vi "Find Intersections of Fitted Line with Universal Circle.vi"(8 "Error In":errorcluster, 10 "Complex Coordinates":cluster{"g Array":sgl[], "s Array":sgl[]}, 11 "Phasor Array":T1[](array[typedef]) {"s" format="%#_4g"; "g" format="%#_4g"}) -> (0 "Error Out":errorcluster, 1 "mu-":dbl format="%#_4g", 2 "Intersection 2":cluster{"x":dbl, "y":dbl} {"x" format="%#_4g"; "y" format="%#_4g"}, 3 "Intersection 1":cluster{"x":dbl, "y":dbl} {"x" format="%#_4g"; "y" format="%#_4g"}, 5 "mu+":dbl format="%#_4g")   [LabVIEW 2019]
uses:
  Phasor (g, s).ctl
  <vilib>/Utility/error.llb/DialogType.ctl
  <vilib>/Analysis/6fits.llb/Curve Fitting Criteria.ctl
  <vilib>/Analysis/NI_AALPro.lvlib
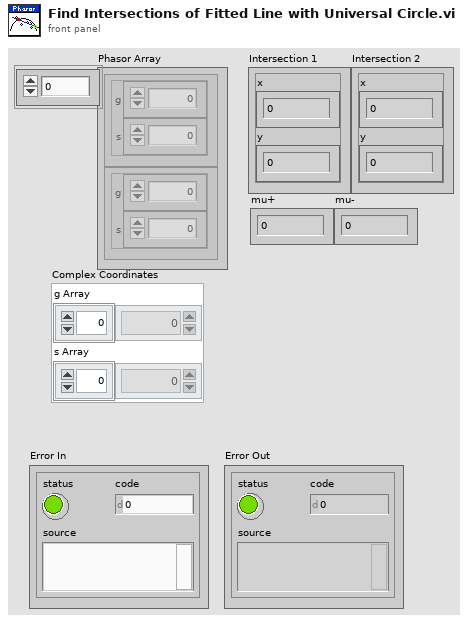
[diagram p1: front panel]
types:
  T1 = typedef "Phasor (g, s).ctl" = cluster{"g":dbl, "s":dbl}
  T2 = typedef "DialogType.ctl" = u16
  T3 = typedef "NI_AALPro.lvlib/Curve Fitting Criteria.ctl" = u16
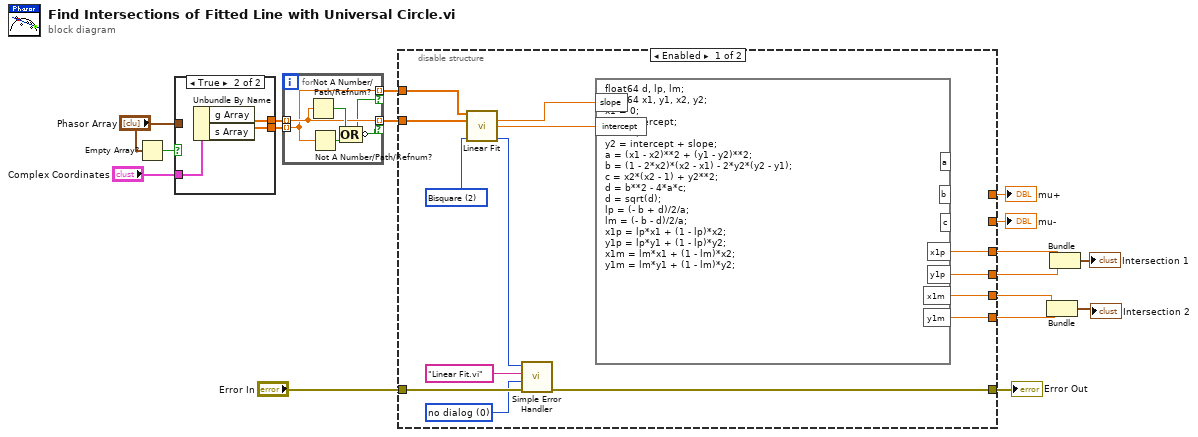
[diagram p0: block diagram]
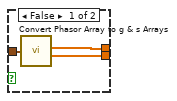
[diagram p2: hidden frame]
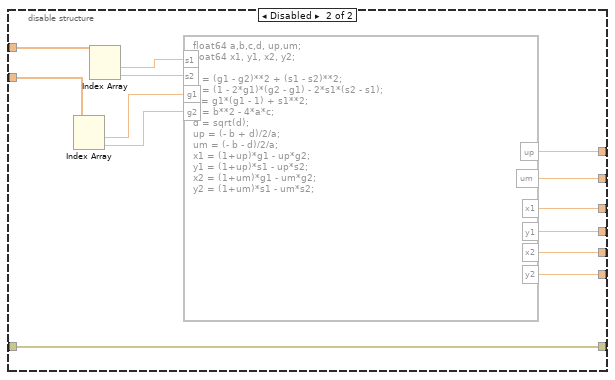
[diagram p3: hidden frame]
diagram:
  n1 = Empty Array?(array="Phasor Array") -> (empty?=w2:bool)
  n2 = case shown="True" w2 {
    tunnel: [w20 w22] -> w9
    tunnel: [w19 w21] -> w8
    tunnel: "Phasor Array" -> [w18 _]
    tunnel: "Complex Coordinates" -> [_ w23]
    frame False {
      n3 = call "Convert Phasor Array to g & s Arrays.vi"("Phasor Array"=w18) -> ("g"=w20:dbl[], "s"=w19:dbl[])  [unwired: 8 in]
    }
    frame True {
      n4 = Unbundle By Name(w23) -> ("g Array"=w22:sgl[], "s Array"=w21:sgl[])
    }
  }
  n5 = for {
    tunnel: w9 -> [w26] mode=indexing
    tunnel: w8 -> [w25] mode=indexing
    tunnel: [w26] -> w7 mode=indexing if=w24
    tunnel: [w25] -> w6 mode=indexing if=w24
    n6 = Not A Number/Path/Refnum?(number/path/refnum=w26) -> (NaN/Path/Refnum?=w27:bool)
    n7 = Not A Number/Path/Refnum?(number/path/refnum=w25) -> (NaN/Path/Refnum?=w28:bool)
    n8 = Compound Arithmetic op=OR(w27, w28) -> (invert w24:bool)
  }
  n9 = disable-structure shown="Enabled" {
    disable-tunnel: [w42 w53] -> w17
    disable-tunnel: [w41 w52] -> w16
    disable-tunnel: [w40 w51] -> w14
    disable-tunnel: [w39 w50] -> w13
    disable-tunnel: "Error In" -> [w38 w49]
    disable-tunnel: [w34 w49] -> w10
    disable-tunnel: w7 -> [w30 w54]
    disable-tunnel: w6 -> [w29 w55]
    disable-tunnel: [_ w48] -> w5
    disable-tunnel: [_ w47] -> w4
    frame Enabled {
      w31 = T2 0 items=["no dialog", "OK message", "continue or stop message", "OK message + warnings", "continue/stop + warnings"] ("type of dialog (OK msg:1)")
      w37 = T3 2 items=["Least Square", "Least Absolute Residual", "Bisquare"] ("method")
      n10 = call <vilib>:"Linear Fit.vi"("Y"=w29, "X"=w30, "method"=w37) -> ("slope"=w36:dbl, "intercept"=w35:dbl, "error"=w33:i32)  [unwired: 8 in, 2 out]
      n11 = call <vilib>:"Simple Error Handler.vi"("error code (no error:0)"=w33, "error source (\" \")"="Linear Fit.vi" ("error source (\" \")"), "type of dialog (OK msg:1)"=w31, "error in (no error)"=w38) -> ("error out"=w34:errorcluster)  [unwired: 1 in, 4 out]
      n12 = formula code="float64 d, lp, lm;\nfloat64 x1, y1, x2, y2;\nx1 = 0;\ny1 = intercept;\nx2 = 1;\ny2 = intercept + slope;\na = (x1 - x2)**2 + (y1 - y2)**2;\nb = (1 - 2*x2)*(x2 - x1) - 2*y2*(y2 - y1);\nc = x2*(x2 - 1) + y2**2;\nd = b**2 - 4*a*c;\nd = sqrt(d);\nlp = (- b + d)/2/a;\nlm = (- b - d)/2/a;\nx1p = lp*x1 + (1 - lp)*x2;\ny1p = lp*y1 + (1 - lp)*y2;\nx1m = lm*x1 + (1 - lm)*x2;\ny1m = lm*y1 + (1 - lm)*y2;"("slope"=w36, "intercept"=w35) -> ("x1p"=w42:dbl, "x1m"=w40:dbl, "y1p"=w41:dbl, "y1m"=w39:dbl)  [unwired: 3 out]
    }
    frame Disabled {
      n13 = Index Array(array=w54) -> (element #1=w44:dbl, element #2=w43:dbl)  [unwired: 2 in]
      n14 = Index Array(array=w55) -> (element #1=w46:dbl, element #2=w45:dbl)  [unwired: 2 in]
      n15 = formula code="float64 a,b,c,d, up,um;\nfloat64 x1, y1, x2, y2;\n\na = (g1 - g2)**2 + (s1 - s2)**2;\nb = (1 - 2*g1)*(g2 - g1) - 2*s1*(s2 - s1);\nc = g1*(g1 - 1) + s1**2;\nd = b**2 - 4*a*c;\nd = sqrt(d);\nup = (- b + d)/2/a;\num = (- b - d)/2/a;\nx1 = (1+up)*g1 - up*g2;\ny1 = (1+up)*s1 - up*s2;\nx2 = (1+um)*g1 - um*g2;\ny2 = (1+um)*s1 - um*s2;"("s1"=w46, "s2"=w45, "g1"=w44, "g2"=w43) -> ("x1"=w53:dbl, "x2"=w51:dbl, "y1"=w52:dbl, "y2"=w50:dbl, "up"=w48:dbl, "um"=w47:dbl)
    }
  }
  "Error Out" <- w10
  "mu+" <- w5
  "mu-" <- w4
  n16 = Bundle("x1m"=w14, "y1m"=w13) -> (→"Intersection 2":cluster{"x1m":dbl, "y1m":dbl})  [unwired: 1 in]
  n17 = Bundle("x1p"=w17, "y1p"=w16) -> (→"Intersection 1":cluster{"x1p":dbl, "y1p":dbl})  [unwired: 1 in]
